vi "GetCarType.vi"(8 "Error In":errorcluster, 11 "reference in":refnum<class "Sedan.lvclass">) -> (0 "Error Out":errorcluster, 2 "Car Type":string, 3 "reference out":refnum<class "Sedan.lvclass">)   [LabVIEW 2024, in "Sedan.lvclass"]
uses:
  Sedan.lvclass
  Sedan.lvclass/Sedan.ctl
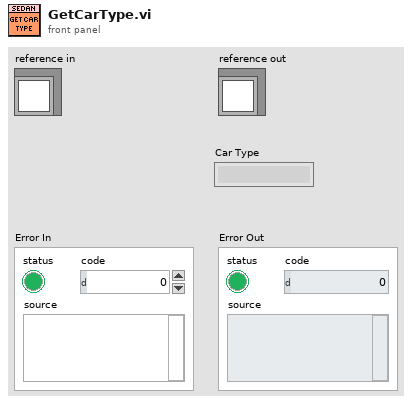
[diagram p1: front panel]
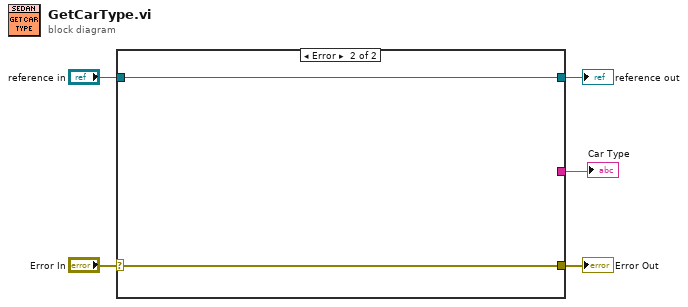
[diagram p0: block diagram]
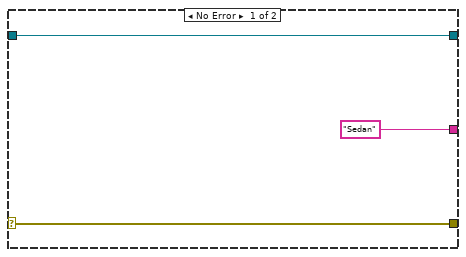
[diagram p2: hidden frame]
diagram:
  n1 = case shown="Error" "Error In" {
    selector: "Error In" -> [w7 w10]
    tunnel: [w7 w10] -> w4
    tunnel: [w8 w9] -> w2
    tunnel: "reference in" -> [w8 w9]
    tunnel: ["Sedan" ("Car Type") _] -> w1
    frame No Error {
    }
    frame Error {
    }
  }
  "Error Out" <- w4
  "reference out" <- w2
  "Car Type" <- w1
